vi "SaveLogFile.vi"(4 "logs in":string[][](table)=[["0.000000", "0.000000", "0.000000"], ["100.000000", "0.000000", "0.000000"], ["200.000000", "0.000000", "0.000000"], ["300.000000", "0.000000", "0.000000"], ["400.000000", "0.000000", "0.000000"]] caption="Loop variable", 8 "error in":errorcluster, 10 "name or relative path":string, 11 "saving folder":path=path "D:/Data/Mai/test target/logfile") -> (0 "error out":errorcluster)   [LabVIEW 2018, in "RW_Protocols.lvlib"]
uses:
  RW_Protocols.lvlib
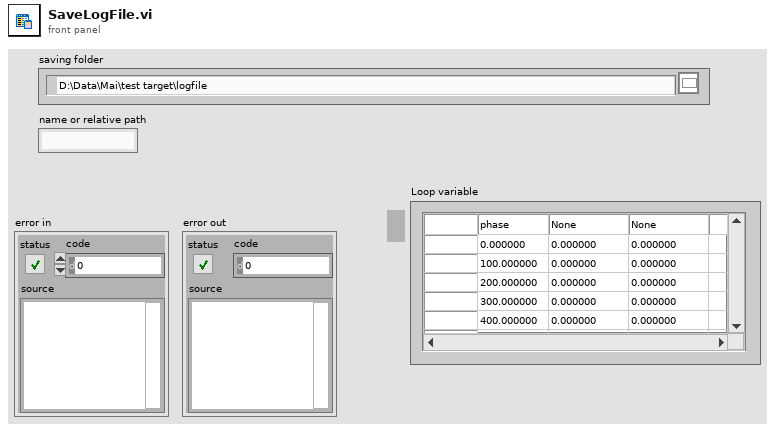
[diagram p1: front panel]
types:
  T1 = enum16{"open", "replace", "create", "open or create", "replace or create", "replace or create with confirmation"}
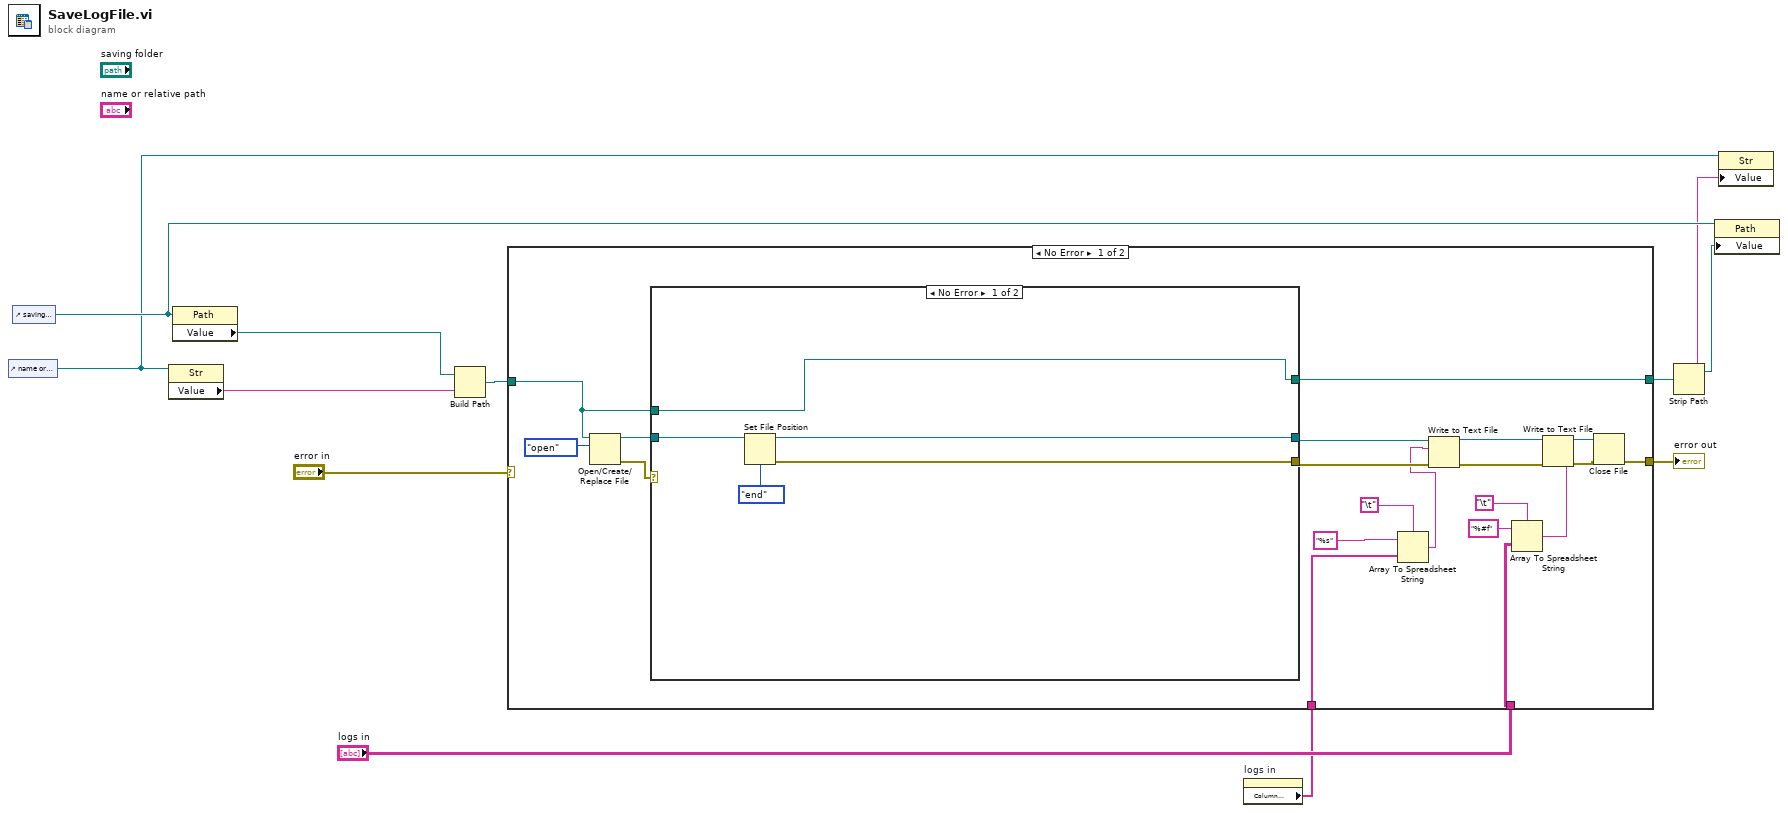
[diagram p0: block diagram]
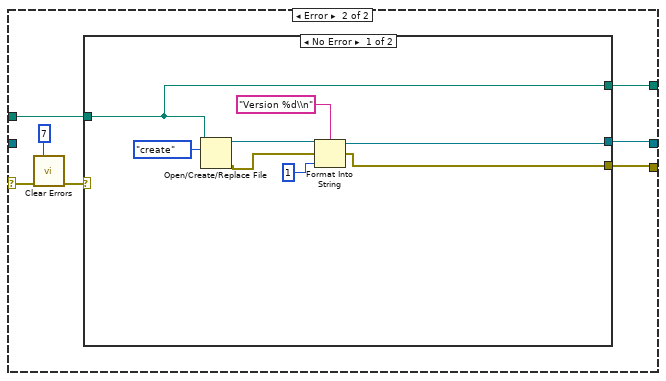
[diagram p2: hidden frame]
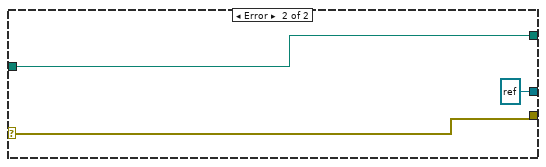
[diagram p3: hidden frame]
diagram:
  n1 = control-ref of="name or relative path"() -> (w6:refnum<vi>)
  n2 = control-ref of="saving folder"() -> (w9:refnum<vi>)
  n3 = property class="Str"(reference=w6) -> ("Value"=w7:string)  [unwired: 1 in, 2 out]
  n4 = property class="Path"(reference=w9) -> ("Value"=w10:path)  [unwired: 1 in, 2 out]
  n5 = Build Path(base path=w10, name or relative path=w7) -> (appended path=w3:path)
  n6 = property on="logs in" class="Tbl (strict)"() -> ("Column Headers[]"=w1:string[])  [unwired: 2 in, 2 out]
  n7 = case shown="No Error" "error in" {
    selector: "error in" -> [_ w57]
    tunnel: [w28 w57] -> w12
    tunnel: [w31 w56] -> w11
    tunnel: w3 -> [w27 w56]
    tunnel: "logs in" -> [w21 _]
    tunnel: w1 -> [w18 _]
    frame No Error {
      n8 = Open/Create/Replace File(file path (use dialog)=w27, operation (0:open)=T1."open") -> (refnum out=w30:refnum<file>, error out=w29:errorcluster)  [unwired: 4 in, 1 out]
      n9 = case shown="No Error" w29 {
        selector: w29 -> [_ w43]
        tunnel: [w35 w40] -> w31
        tunnel: w30 -> [w36 _]
        tunnel: w27 -> [w35 w44]
        tunnel: [w33 w38] -> w14
        tunnel: [w34 w39] -> w17
        frame No Error {
          n10 = Set File Position(refnum=w36, from (0:start)=enum16{"start", "end", "current"}."end" ("à partir de (0 : start)")) -> (refnum out=w33:refnum<file>, error out=w34:errorcluster)  [unwired: 2 in]
        }
        frame Error {
          n11 = call <vilib>:"Clear Errors.vi"("error in (no error)"=w43, "specific error code to clear (0: all)"=7) -> ("error out"=w41:errorcluster)  [unwired: 4 in, 1 out]
          n12 = case shown="No Error" w41 {
            selector: w41 -> [_ w54]
            tunnel: w44 -> [w47 w55]
            tunnel: [w47 w55] -> w40
            tunnel: [w45 w54] -> w39
            tunnel: [w46 refnum<file> refnum ("refnum out")] -> w38
            frame No Error {
              n13 = Open/Create/Replace File(file path (use dialog)=w47, operation (0:open)=T1."create") -> (refnum out=w48:refnum<file>, error out=w49:errorcluster)  [unwired: 4 in, 1 out]
              n14 = Format Into String ("Format Into File")(format string="Version %d\\n", initial string=w48, error in=w49, u32 1 ("input 1")) -> (resulting string=w46:refnum<file>, error out=w45:errorcluster)
            }
            frame Error {
            }
          }
        }
      }
      n15 = Array To Spreadsheet String(delimiter (Tab)="\t", array=w18, 3:"%s" ("format string")) -> (spreadsheet string=w13:string)
      n16 = Write to Text File(file (use dialog)=w14, text=w13, error in=w17) -> (refnum out=w15:refnum<file>, error out=w16:errorcluster)  [unwired: 1 in, 1 out]
      n17 = Array To Spreadsheet String(delimiter (Tab)="\t", array=w21, 3:"%#f" ("format string")) -> (spreadsheet string=w22:string)
      n18 = Write to Text File(file (use dialog)=w15, text=w22, error in=w16) -> (refnum out=w23:refnum<file>, error out=w24:errorcluster)  [unwired: 1 in, 1 out]
      n19 = Close File(refnum=w23, error in=w24) -> (error out=w28:errorcluster)  [unwired: 1 out]
    }
    frame Error {
    }
  }
  "error out" <- w12
  n20 = Strip Path(path=w11) -> (stripped path=w8:path, name=w5:string)
  n21 = property class="Path"(reference=w9, "Value"=w8) -> ()  [unwired: 1 in, 2 out]
  n22 = property class="Str"(reference=w6, "Value"=w5) -> ()  [unwired: 1 in, 2 out]
